vi "Teleop_Calc_Inlet.vi"(11 "Teleop Local Data in":T1) -> (3 "Teleop Local Data out":T1)   [LabVIEW 2016]
uses:
  Typedefs/typedef_cluster_Teleop Local Data.ctl
  Typedefs/typedef_enum_Joystick Buttons.ctl
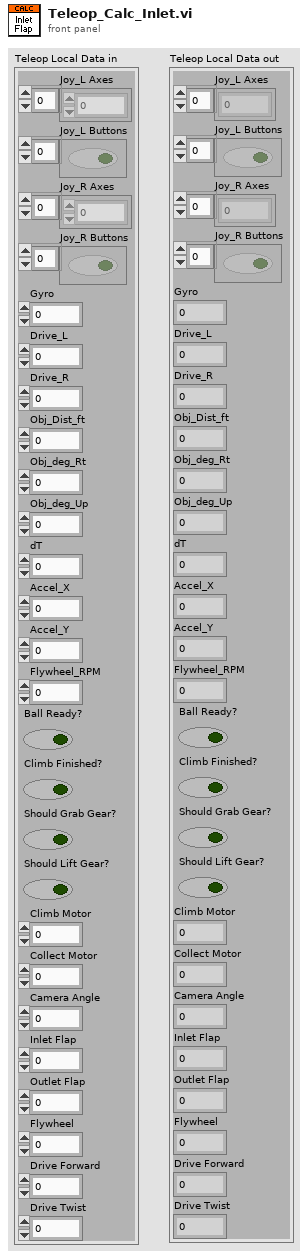
[diagram p1: front panel]
types:
  T1 = typedef "typedef_cluster_Teleop Local Data.ctl" = cluster{"Joy_L Axes":dbl[], "Joy_L Buttons":bool[], "Joy_R Axes":dbl[], "Joy_R Buttons":bool[], "Gyro":dbl, "Drive_L":i32, "Drive_R":i32, "Obj_Dist_ft":dbl, "Obj_deg_Rt":dbl, "Obj_deg_Up":dbl, "dT":dbl, "Accel_X":dbl, "Accel_Y":dbl, "Flywheel_RPM":dbl, "Ball Ready?":bool, "Climb Finished?":bool, "Should Grab Gear?":bool, "Should Lift Gear?":bool, "Climb Motor":dbl, "Collect Motor":dbl, "Camera Angle":dbl, "Inlet Flap":dbl, "Outlet Flap":dbl, "Flywheel":dbl, "Drive Forward":dbl, "Drive Twist":dbl}
  T2 = typedef "typedef_enum_Joystick Buttons.ctl" = enum16{"Trigger", "Thumb", "Top3", "Top4", "Top5", "Top6", "Low7", "Low8", "Low9", "Low10", "Low11", "Low12", "Hat0", "Hat1", "Hat2", "Hat3", "Hat4", "Hat5", "Hat6", "Hat7", "Hat8"}
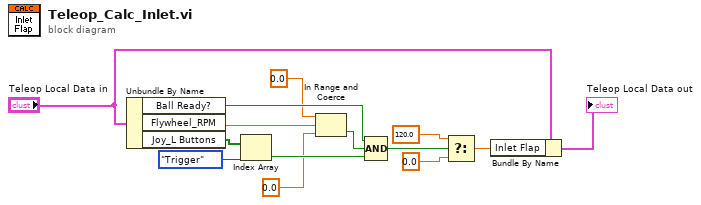
[diagram p0: block diagram]
diagram:
  n1 = Unbundle By Name("Teleop Local Data in") -> ("Ball Ready?"=w3:bool, "Flywheel_RPM"=w7:dbl, "Joy_L Buttons"=w8:bool[])
  n2 = Index Array(array=w8, index=typedef_enum_Joystick_Buttons."Trigger" ("Joystick Buttons")) -> (element=w5:bool)
  n3 = In Range and Coerce(upper limit=0.0, x=w7, lower limit=0.0) -> (In Range?=w4:bool)  [unwired: 1 out]
  n4 = Compound Arithmetic op=AND(w3, w4, w5) -> (w6:bool)
  n5 = Select(t=120.0, s=w6, f=0.0 ("Position")) -> (s? t:f=w11:dbl)
  n6 = Bundle By Name(cluster="Teleop Local Data in", "Inlet Flap"=w11) -> (→"Teleop Local Data out":T1)
